vi "Exo2.vi"() -> ()   [LabVIEW 2018]
panel:
  out "Led":bool
  in  "Bouton 3":i8(knob) min=0 max=9 scale=0.0..10.0
  in  "Bouton 2":i8(knob) min=0 max=9 scale=0.0..10.0
  in  "Bouton 1":i8(knob) min=0 max=9 scale=0.0..10.0
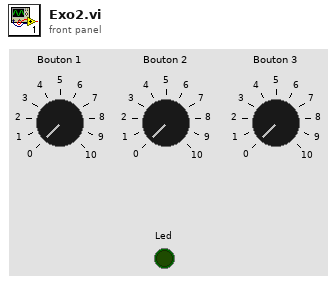
[diagram p1: front panel]
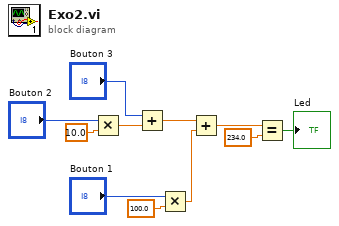
[diagram p0: block diagram]
diagram:
  n1 = Multiply(x="Bouton 2", y=10.0 ("x")) -> (x*y=w9:dbl)
  n2 = Add(x="Bouton 3", y=w9) -> (x+y=w8:dbl)
  n3 = Multiply(x="Bouton 1", y=100.0) -> (x*y=w6:dbl)
  n4 = Add(x=w8, y=w6) -> (x+y=w5:dbl)
  n5 = Equal?(x=w5, y=234.0) -> (x = y?=→"Led":bool)
